vi "read_data.vi"(8 "error in (no error)":errorcluster, 11 "GenericDAQ in":refnum<class "GenericDAQ.lvclass">) -> (0 "error out":errorcluster, 2 "finished?":bool, 3 "GenericDAQ out":refnum<class "GenericDAQ.lvclass">, 4 "buffer overflow?":bool)   [LabVIEW 2010, in "GenericDAQ.lvclass"]
uses:
  GenericDAQ.lvclass
  GenericDAQ.lvclass/GenericDAQ.ctl
  common/classes/GenericComponent/GenericComponent/class_data.vi
  common/classes/ErrorController/ErrorController/class_data.vi
  common/classes/ErrorController/ErrorController/ErrorController.lvclass
  common/classes/GenericComponent/GenericComponent/GenericComponent.lvclass
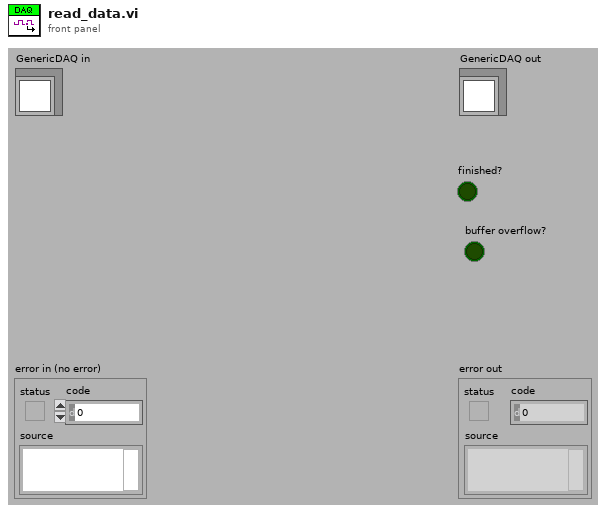
[diagram p1: front panel]
types:
  T1 = typedef "pixel_raw_data_array.ctl" = dbl[][]
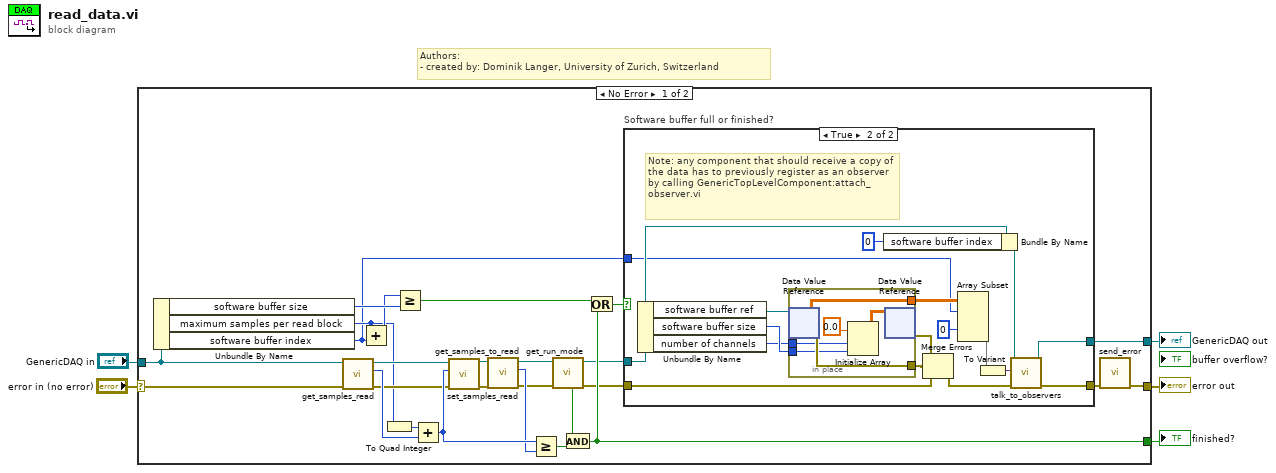
[diagram p0: block diagram]
diagram:
  # "Authors: \n- created by: Dominik Langer, University of Zurich, Switzerland"
  n1 = case shown="No Error" "error in (no error)" {
    selector: "error in (no error)" -> [w31 w58]
    tunnel: [w12 w58] -> w4
    tunnel: [w23 w57] -> w2
    tunnel: "GenericDAQ in" -> [w14 w57]
    tunnel: [w21 _] -> w1
    frame No Error {
      n2 = Unbundle By Name(w14) -> ("software buffer size"=w22:i32, "maximum samples per read block"=w7:i32, "software buffer index"=w6:i32)
      n3 = call-dynamic "get_samples_read.vi"("error in (no error)"=w31, "GenericDAQ.lvclass in"=w14) -> ("error out"=w10:errorcluster, "samples read"=w26:i64, "GenericDAQ.lvclass out"=w9:refnum<class "GenericDAQ.lvclass">)  [unwired: 7 out]
      n4 = Add(x=w7, y=w6) -> (x+y=w8:i32)
      n5 = To Quad Integer(1:w7) -> (0:w27:i64)
      n6 = Greater Or Equal?(x=w8, y=w22) -> (x >= y?=w20:bool)
      n7 = Add(x=w27, y=w26) -> (x+y=w28:i64)
      n8 = call-dynamic "set_samples_read.vi"("error in (no error)"=w10, "samples read"=w28, "GenericDAQ.lvclass in"=w9) -> ("error out"=w30:errorcluster, "GenericDAQ.lvclass out"=w29:refnum<class "GenericDAQ.lvclass">)  [unwired: 7 out]
      n9 = call-dynamic "get_samples_to_read.vi"("error in (no error)"=w30, "GenericDAQ.lvclass in"=w29) -> ("error out"=w18:errorcluster, "samples to read"=w25:i64, "GenericDAQ.lvclass out"=w16:refnum<class "GenericDAQ.lvclass">)  [unwired: 7 out]
      n10 = Greater Or Equal?(x=w28, y=w25) -> (x >= y?=w24:bool)
      n11 = call "get_run_mode.vi"("error in (no error)"=w18, "GenericPlugin in"=w16) -> ("error out"=w17:errorcluster, "GenericPlugin out"=w13:refnum<class "GenericDAQ.lvclass">, "is NOT free run?"=w15:bool)  [unwired: 5 in, 2 out]
      n12 = And(x=w15, y=w24) -> (x .and. y?=w21:bool)
      n13 = Or(x=w20, y=w21) -> (x .or. y?=w19:bool)
      n14 = case "Software buffer full or finished?" shown="True" w19 {
        tunnel: w17 -> [w33 w42]
        tunnel: [w33 w45] -> w11
        tunnel: [w32 w41] -> w23
        tunnel: w13 -> [w32 w40]
        tunnel: w6 -> [_ w35]
        frame False {
        }
        frame True {
          # "Note: any component that should receive a copy of the data has to previously register as an observer by calling GenericTopLevelComponent:attach_observer.vi"
          n15 = Unbundle By Name(w40) -> ("software buffer ref"=w49:refnum<data-value>, "software buffer size"=w44:i32, "number of channels"=w43:i32)
          n16 = in-place {
            in-place-border: [w56] -> w47
            in-place-border: [w55] -> w37
            in-place-border: w44 -> [w53]
            in-place-border: w43 -> [w52]
            n17 = in-place-dvr #1(w49) -> (w55:T1, w56:errorcluster)
            n18 = Initialize Array(0.0, w52, w53) -> (w51:dbl[][])
            n19 = in-place-dvr #1(w51) -> (w48:errorcluster)  [unwired: 1 out]
          }
          n20 = Bundle By Name(cluster=w40, "software buffer index"=0) -> (w39:refnum<class "GenericDAQ.lvclass">)
          n21 = Merge Errors(w48, w47, w42) -> (w46:errorcluster)
          n22 = Array Subset(array=w37, index (col)=0 ("index"), length (col)=w35) -> (w34:T1)  [unwired: 2 in]
          n23 = To Variant(anything=w34) -> (Variant=w50:variant)
          n24 = call-dynamic "talk_to_observers.vi"("error in (no error)"=w46, "data"=w50, "GenericToplevelComponent in"=w39) -> ("error out"=w45:errorcluster, "GenericToplevelComponent out"=w41:refnum<class "GenericDAQ.lvclass">)  [unwired: 7 in]
        }
      }
      n25 = call "send_error.vi"("error in (no error)"=w11) -> ("error out"=w12:errorcluster)  [unwired: 10 in]
    }
    frame Error {
    }
  }
  "error out" <- w4
  "GenericDAQ out" <- w2
  "finished?" <- w1
